vi "Handle Encoder Failure.vi"(6 "PID gains":T1={"proportional gain (Kc)"=1.0, "integral time (Ti, min)"=0.01, "derivative time (Td, min)"=0.0} {"derivative time (Td, min)" format="%.3f"; "integral time (Ti, min)" format="%.3f"; "proportional gain (Kc)" format="%.3f"}, 7 "Output Range":cluster{"output high":dbl, "output low":dbl}={"output high"=100.0, "output low"=-100.0} {"output low" format="%.2f"; "output high" format="%.2f"}, 8 "Encoder Failure":bool, 9 "Loop Time":dbl, 10 "Desired RPM":dbl, 11 "Current RPM":dbl) -> (1 "Encoder Failure Out":bool, 2 "Motor Output":dbl)   [LabVIEW 2012]
uses:
  <vilib>/addons/control/pid/pid.llb/PID (DBL).vi
  <vilib>/addons/control/pid/NI_PID_pid.lvlib
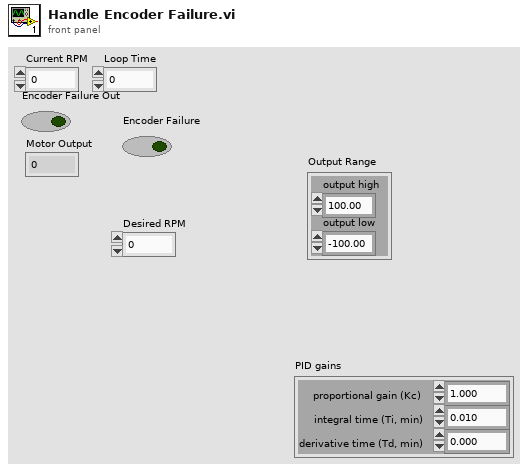
[diagram p1: front panel]
types:
  T1 = cluster{"proportional gain (Kc)":dbl, "integral time (Ti, min)":dbl, "derivative time (Td, min)":dbl}
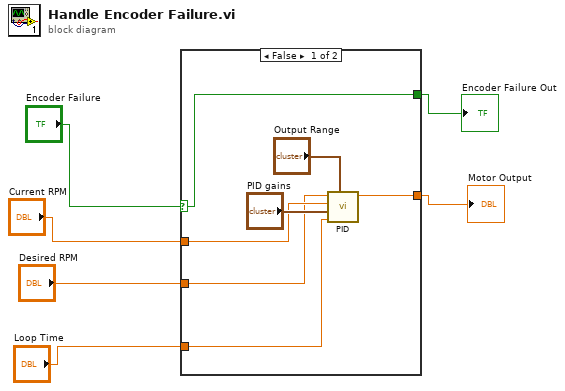
[diagram p0: block diagram]
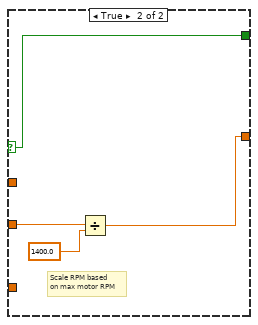
[diagram p2: hidden frame]
diagram:
  n1 = case shown="False" "Encoder Failure" {
    selector: "Encoder Failure" -> [w7 w17]
    tunnel: "Loop Time" -> [w9 _]
    tunnel: "Desired RPM" -> [w10 w16]
    tunnel: "Current RPM" -> [w11 _]
    tunnel: [w8 w14] -> w1
    tunnel: [w7 w17] -> w2
    frame False {
      n2 = call-poly <vilib>:"PID.vi"("output range"="Output Range", "dt (s)"=w9, "PID gains"="PID gains", "process variable"=w11, "setpoint"=w10) -> ("output"=w8:dbl)  [unwired: 5 in, 1 out]
    }
    frame True {
      # "Scale RPM based\non max motor RPM"
      n3 = Divide(x=w16, y=1400.0) -> (x/y=w14:dbl)
    }
  }
  "Encoder Failure Out" <- w2
  "Motor Output" <- w1
